vi "测试信号灯成员类.vi"() -> ()   [LabVIEW 2017]
panel:
  out "红":bool
  out "黄":bool
  out "绿":bool
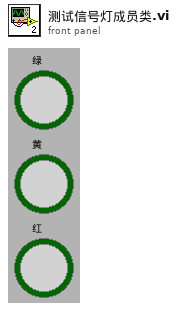
[diagram p1: front panel]
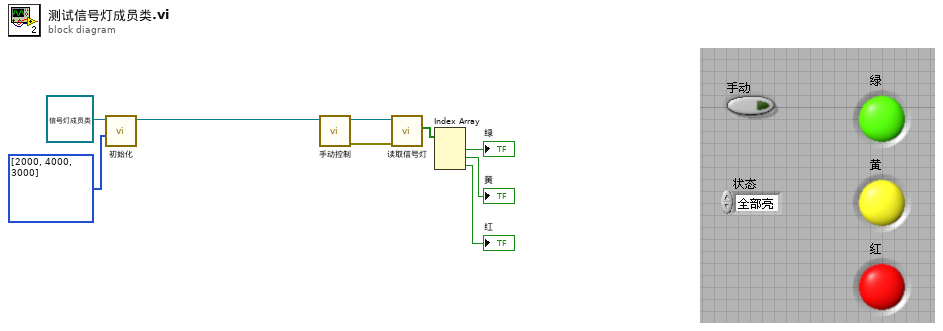
[diagram p0: block diagram]
diagram:
  n1 = call "初始化.vi"("设定时间"=u32[] [2000, 4000, 3000], "信号灯成员类 输入"=refnum<class "信号灯成员类.lvclass"> refnum ("信号灯成员类.lvclass")) -> ("信号灯成员类 输出"=w8:refnum<class "信号灯成员类.lvclass">)  [unwired: 1 in, 8 out]
  n2 = call "手动控制.vi"("信号灯成员类 输入"=w8) -> ("error out"=w4:errorcluster, "信号灯成员类 输出"=w5:refnum<class "信号灯成员类.lvclass">)  [unwired: 3 in, 6 out]
  n3 = call "读取信号灯.vi"("error in (no error)"=w4, "信号灯成员类.lvclass输入"=w5) -> ("信号灯"=w6:bool[])  [unwired: 9 out]
  n4 = Index Array(array=w6) -> (element #1=→"绿":bool, element #2=→"黄":bool, element #3=→"红":bool)  [unwired: 3 in]
